vi "DAQ_NetworkConfigs.vi"(8 "error in":errorcluster, 10 "StreamCluster_TypeDef":T1={"DAQ"={"ManagmentRate_Hz"=1000, "StreamRate_Hz"=10, "refDesArray"=[], "StreamRate_ms"=0, "ManagmentRate_ms"=1000}, "Modules"=[]}, 11 "DOM document in":refnum<k20>) -> (0 "error out":errorcluster, 2 "StreamCluster_TypeDef 2":T1={"DAQ"={"ManagmentRate_Hz"=1000, "StreamRate_Hz"=10, "refDesArray"=[], "StreamRate_ms"=0, "ManagmentRate_ms"=1000}, "Modules"=[]}, 3 "DOM document out":refnum<k20>)   [LabVIEW 2024]
uses:
  <vilib>/xml/NI_XML.lvlib
  <vilib>/xml/Close Reference(Node).vi
  Control/StreamCluster_TypeDef.ctl
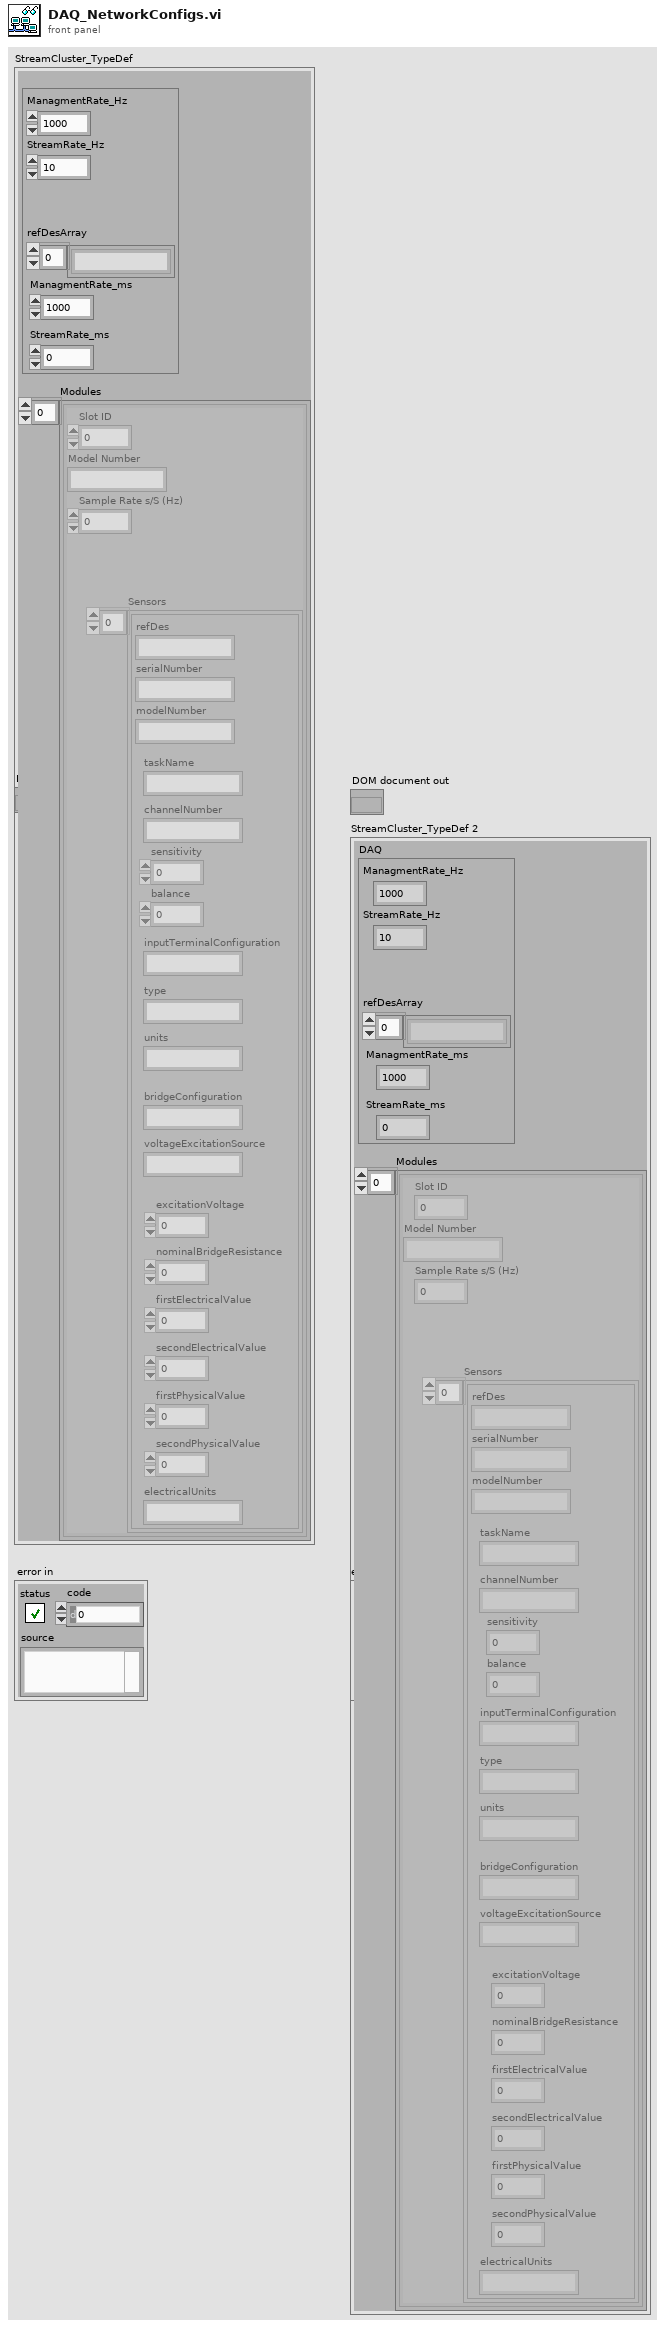
[diagram p1: front panel]
types:
  T1 = typedef "StreamCluster_TypeDef.ctl" = cluster{"DAQ":cluster{"ManagmentRate_Hz":i32, "StreamRate_Hz":i32, "refDesArray":string[], "StreamRate_ms":i32, "ManagmentRate_ms":i32}, "Modules":cluster{"Slot ID":i32, "Model Number":string, "Sample Rate s/S (Hz)":dbl, "Sensors":cluster{"refDes":string, "serialNumber":string, "modelNumber":string, "units":string, "balance":dbl, "sensitivity":dbl, "type":string, "inputTerminalConfiguration":string, "channelNumber":string, "taskName":string, "bridgeConfiguration":string, "excitationVoltage":dbl, "voltageExcitationSource":string, "nominalBridgeResistance":dbl, "firstElectricalValue":dbl, "secondElectricalValue":dbl, "firstPhysicalValue":dbl, "secondPhysicalValue":dbl, "electricalUnits":string}[]}[]}
  T2 = cluster{"[0]":string, "[1]":string, "[2]":string, "[3]":string, "[4]":string, "[5]":string, "[6]":string, "[7]":string, "[8]":string}
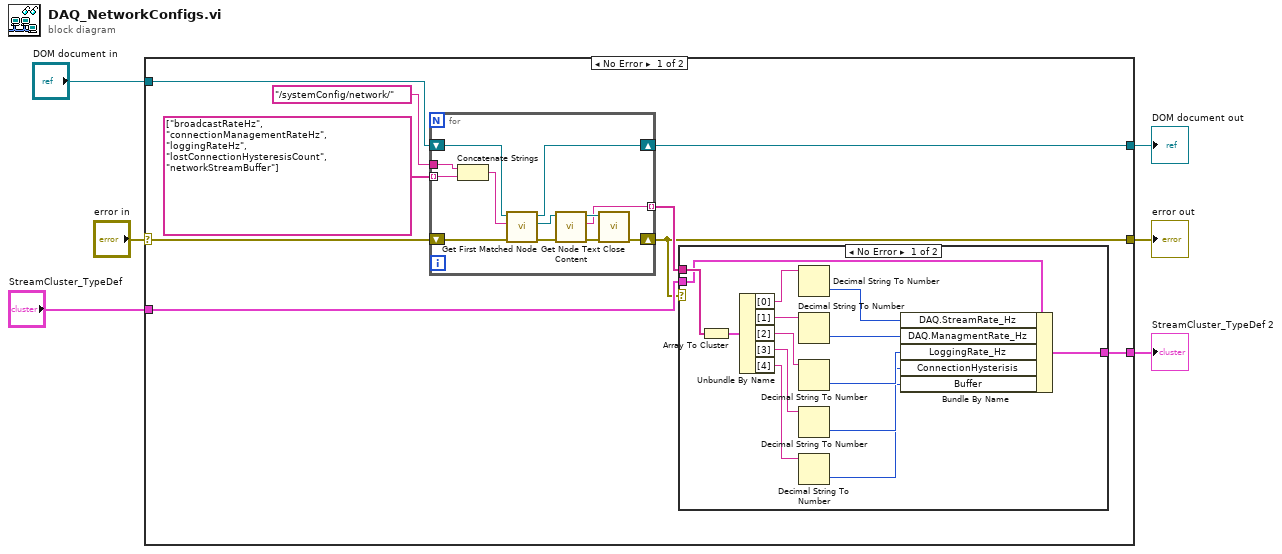
[diagram p0: block diagram]
diagram:
  n1 = case shown="No Error" "error in" {
    selector: "error in" -> [w13 w45]
    tunnel: [w7 w45] -> w5
    tunnel: "DOM document in" -> [w12 w44]
    tunnel: [w11 w44] -> w3
    tunnel: [w8 w43] -> w2
    tunnel: "StreamCluster_TypeDef" -> [w9 w43]
    frame No Error {
      n2 = for {
        tunnel: "/systemConfig/network/" ("XPath expression") -> [w38]
        tunnel: string[] ["broadcastRateHz", "connectionManagementRateHz", "loggingRateHz", "lostConnectionHysteresisCount", "networkStreamBuffer"] -> [w37] mode=indexing
        shift-right: [w33] -> w11
        shift-left: w12 -> [w39]
        shift-right: [w32] -> w7
        shift-left: w13 -> [w40]
        tunnel: [w31] -> w10 mode=indexing
        n3 = Concatenate Strings(w38, w37) -> (w36:string)
        n4 = call <vilib>:"Get First Matched Node.vi"("error in (no error)"=w40, "XPath expression"=w36, "node in"=w39) -> ("error out"=w41:errorcluster, "node result"=w42:refnum<k20>, "node out"=w33:refnum<k20>)  [unwired: 6 in]
        n5 = call <vilib>:"Get Node Text Content.vi"("error in (no error)"=w41, "node in"=w42) -> ("error out"=w35:errorcluster, "node text"=w31:string, "node out"=w34:refnum<k20>)  [unwired: 7 in]
        n6 = call-poly <vilib>:"Close.vi"("error in (no error)"=w35, "node"=w34) -> ("error out"=w32:errorcluster)  [unwired: 7 out]
      }
      n7 = case shown="No Error" w7 {
        tunnel: w10 -> [w29 _]
        tunnel: w9 -> [w27 w30]
        tunnel: [w26 w30] -> w8
        frame No Error {
          n8 = Array To Cluster(array=w29) -> (cluster=w28:T2)
          n9 = Unbundle By Name(w28) -> ("[0]"=w25:string, "[1]"=w22:string, "[2]"=w20:string, "[3]"=w19:string, "[4]"=w17:string)
          n10 = Decimal String To Number(string=w25) -> (number=w24:i32)  [unwired: 2 in, 1 out]
          n11 = Decimal String To Number(string=w22) -> (number=w23:i32)  [unwired: 2 in, 1 out]
          n12 = Decimal String To Number(string=w20) -> (number=w21:i32)  [unwired: 2 in, 1 out]
          n13 = Decimal String To Number(string=w19) -> (number=w18:i32)  [unwired: 2 in, 1 out]
          n14 = Decimal String To Number(string=w17) -> (number=w16:i32)  [unwired: 2 in, 1 out]
          n15 = Bundle By Name(cluster=w27, "DAQ.StreamRate_Hz"=w24, "DAQ.ManagmentRate_Hz"=w23, "LoggingRate_Hz"=w21, "ConnectionHysterisis"=w18, "Buffer"=w16) -> (w26:T1)
        }
        frame Error {
        }
      }
    }
    frame Error {
    }
  }
  "error out" <- w5
  "DOM document out" <- w3
  "StreamCluster_TypeDef 2" <- w2
